vi "getMasksFloat.vi"(0 "dl in":refnum<class "dl.lvclass">, 5 "numberofDetections":i32, 11 "error in (no error)":errorcluster) -> (4 "dl out":refnum<class "dl.lvclass">, 6 "polySucc":i32, 8 "arrayVrtxFloat":cluster{"x":sgl, "y":sgl}[](array[cluster]), 10 "totalVrtx":i32, 15 "error out":errorcluster)   [LabVIEW 2025, in "dl.lvlib" / "dl.lvclass"]
uses:
  dl.lvclass
  dl.lvclass/dl.ctl
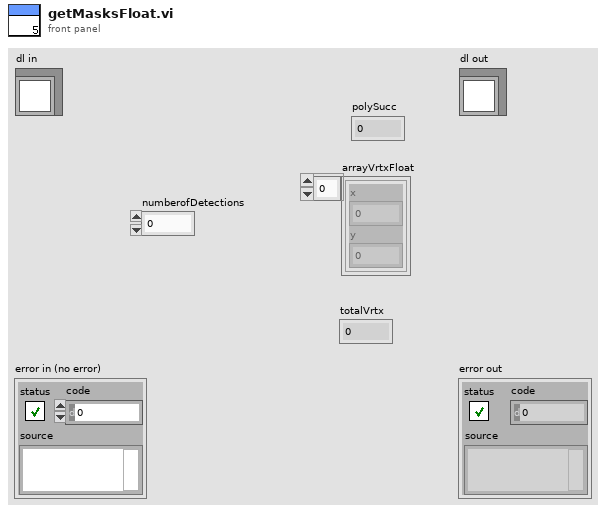
[diagram p1: front panel]
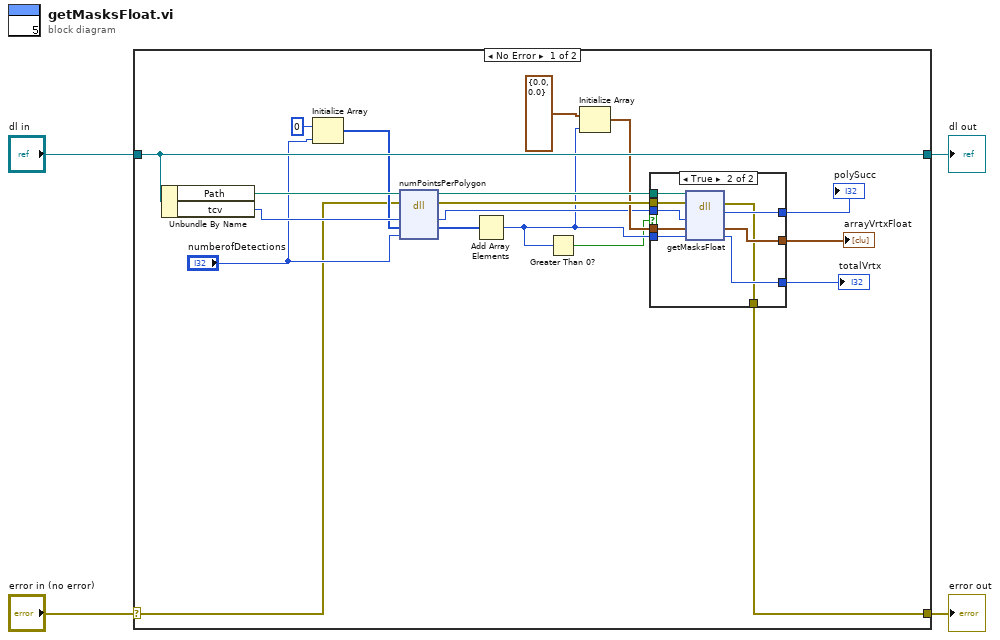
[diagram p0: block diagram]
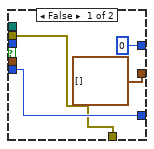
[diagram p2: hidden frame]
diagram:
  n1 = case shown="No Error" "error in (no error)" {
    selector: "error in (no error)" -> [w8 w38]
    tunnel: [w7 w38] -> w3
    tunnel: [w23 w37] -> w1
    tunnel: "dl in" -> [w23 w37]
    frame No Error {
      n2 = Unbundle By Name(w23) -> ("Path"=w22:path, "tcv"=w21:u64)
      n3 = Initialize Array(0 ("element"), "numberofDetections") -> (w18:i32[])
      n4 = dll-call lib="D:/Test/adslvPackageDev/Resources/TCV_Lib.dll" fn="numPointsPerPolygon"(path in=w22, error in=w8, "tcv"=w21, "outCounts"=w18, "numberofDetections"="numberofDetections") -> (path out=w15:path, error out=w14:errorcluster, "tcv"=w12:u64, "outCounts"=w17:i32[])  [unwired: 3 in]
      n5 = Add Array Elements(numeric array=w17) -> (sum=w6:i32)
      n6 = Greater Than 0?(x=w6) -> (x > 0?=w5:bool)
      n7 = Initialize Array(cluster{"x":sgl, "y":sgl} {"x"=0.0, "y"=0.0}, w6) -> (w13:cluster{"x":sgl, "y":sgl}[])
      n8 = case shown="True" w5 {
        tunnel: w15 -> [_ w36]
        tunnel: w14 -> [w24 w35]
        tunnel: w13 -> [_ w34]
        tunnel: w12 -> [_ w33]
        tunnel: w6 -> [w25 w32]
        tunnel: [cluster{"x":sgl, "y":sgl}[] [] ("arrayVrtx") w31] -> w11
        tunnel: [w25 w30] -> w10
        tunnel: [0 ("polySucc") w29] -> w9
        tunnel: [w24 w28] -> w7
        frame False {
        }
        frame True {
          n9 = dll-call lib="D:/Test/adslvPackageDev/Resources/TCV_Lib.dll" fn="getMasksFloat"(path in=w36, error in=w35, "tcv"=w33, "arrayVrtx"=w34, "totalVrtx"=w32) -> (error out=w28:errorcluster, "polySucc"=w29:i32, "arrayVrtx"=w31:cluster{"x":sgl, "y":sgl}[], "totalVrtx"=w30:i32)  [unwired: 2 in, 1 out]
        }
      }
      "arrayVrtxFloat" <- w11
      "totalVrtx" <- w10
      "polySucc" <- w9
    }
    frame Error {
    }
  }
  "error out" <- w3
  "dl out" <- w1
